vi "registerServiceReply.vi"(3 "Service":T1) -> (1 "XML":string)   [LabVIEW 2012, in "ROS_Master.lvclass"]
uses:
  ROS_Master.lvclass
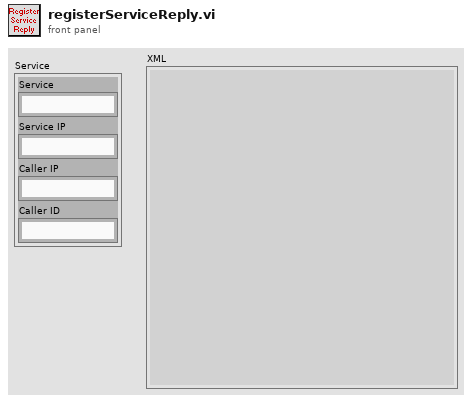
[diagram p1: front panel]
types:
  T1 = cluster{"Service":string, "Service IP":string, "Caller IP":string, "Caller ID":string}
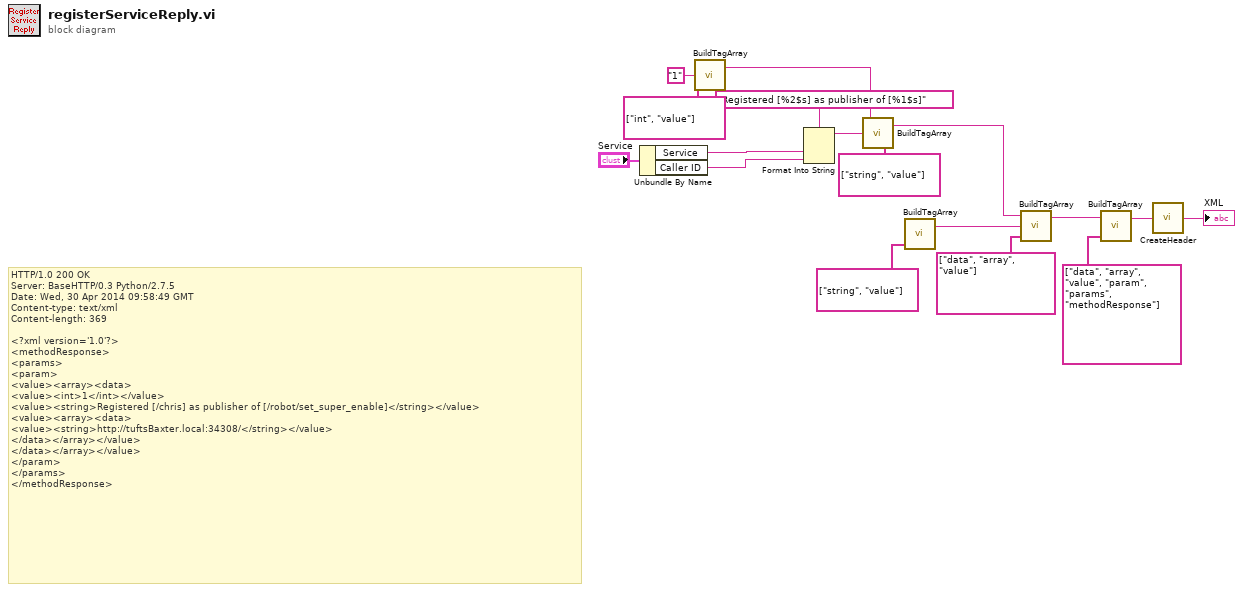
[diagram p0: block diagram]
diagram:
  # "HTTP/1.0 200 OK\nServer: BaseHTTP/0.3 Python/2.7.5\nDate: Wed, 30 Apr 2014 09:58:49 GMT\nContent-type: text/xml\nContent-length: 369\n\n<?xml version='1.0'?>\n<methodResponse>\n<params>\n<param>\n<value><array><data>\n<value><int>1</int></value>\n<value><string>Registered [/chris] as publisher of [/robot/set_super_enable]</string></value>\n<value><array><data>\n<value><string>http://tuftsBaxter.local:34308/</string></value>\n</data></array></value>\n</data></array></value>\n</param>\n</params>\n</methodResponse>"
  n1 = Unbundle By Name("Service") -> ("Service"=w14:string, "Caller ID"=w15:string)
  n2 = call <userlib>:"BuildTagArray.vi"("tags"=string[] ["int", "value"], "value"="1") -> ("string out"=w9:string)  [unwired: 2 in]
  n3 = Format Into String(format string="Registered [%2$s] as publisher of [%1$s]", w14, w15) -> (resulting string=w13:string)  [unwired: 2 in, 1 out]
  n4 = call <userlib>:"BuildTagArray.vi"("tags"=string[] ["string", "value"], "value"=w13, "string in"=w9) -> ("string out"=w8:string)  [unwired: 1 in]
  n5 = call <userlib>:"BuildTagArray.vi"("tags"=string[] ["string", "value"]) -> ("string out"=w1:string)  [unwired: 3 in]
  n6 = call <userlib>:"BuildTagArray.vi"("tags"=string[] ["data", "array", "value"], "value"=w1, "string in"=w8) -> ("string out"=w7:string)  [unwired: 1 in]
  n7 = call <userlib>:"BuildTagArray.vi"("tags"=string[] ["data", "array", "value", "param", "params", "methodResponse"], "value"=w7) -> ("string out"=w5:string)  [unwired: 2 in]
  n8 = call <userlib>:"CreateHeader.vi"("Content"=w5) -> ("XML"=→"XML":string)
